vi "all-quintic-spline-test.vi"(8 "error in (no error)":errorcluster) -> (0 "error out":errorcluster, 3 "ALL TESTS PASSED":bool)   [LabVIEW 2019]
panel:
  out "Test 6":bool
  out "Test 5":bool
  out "Test 4":bool
  out "Test 3B":bool
  out "Test 3A":bool
  out "Test 2":bool
  out "Test 1":bool
  out "Test 0":bool
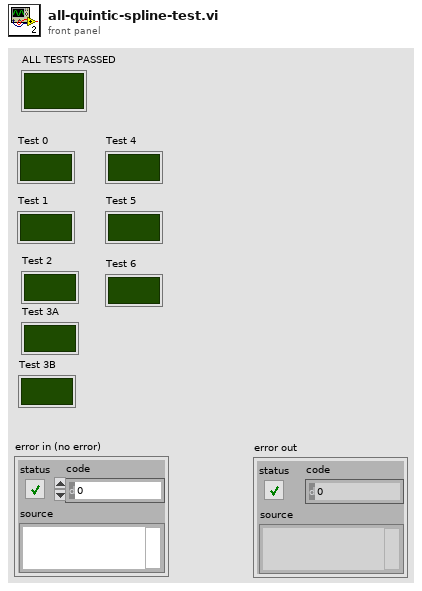
[diagram p1: front panel]
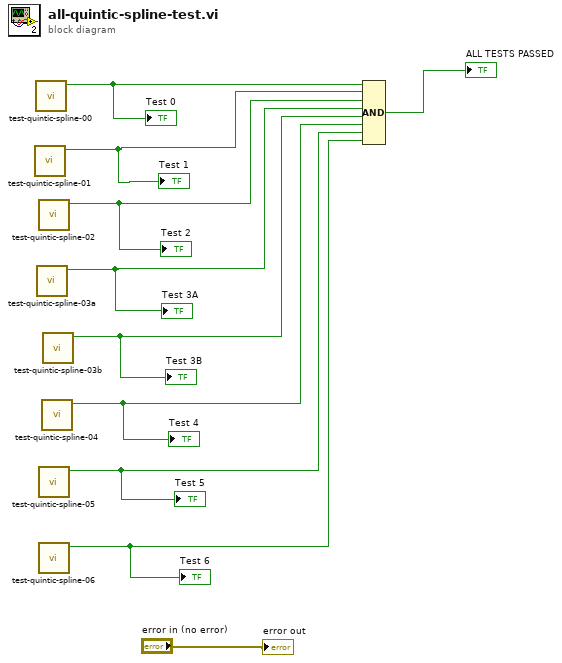
[diagram p0: block diagram]
diagram:
  n1 = call "test-quintic-spline-01.vi"() -> ("Test Passed"=w8:bool)  [unwired: 11 in]
  "Test 1" <- w8
  n2 = call "test-quintic-spline-00.vi"() -> ("Test Passed"=w9:bool)  [unwired: 11 in]
  "Test 0" <- w9
  n3 = call "test-quintic-spline-03a.vi"() -> ("Test Passed"=w5:bool)  [unwired: 11 in]
  "Test 3A" <- w5
  n4 = call "test-quintic-spline-02.vi"() -> ("Test Passed"=w7:bool)  [unwired: 11 in]
  "Test 2" <- w7
  n5 = call "test-quintic-spline-05.vi"() -> ("Test Passed"=w3:bool)  [unwired: 11 in]
  "Test 5" <- w3
  n6 = call "test-quintic-spline-06.vi"() -> ("Test Passed"=w2:bool)  [unwired: 11 in]
  "Test 6" <- w2
  n7 = call "test-quintic-spline-04.vi"() -> ("Test Passed"=w4:bool)  [unwired: 11 in]
  "Test 4" <- w4
  n8 = call "test-quintic-spline-03b.vi"() -> ("Test Passed"=w6:bool)  [unwired: 11 in]
  "Test 3B" <- w6
  n9 = Compound Arithmetic op=AND(w9, w8, w7, w5, w6, w4, w3, w2) -> (→"ALL TESTS PASSED":bool)
  "error out" <- "error in (no error)"
